vi "FTW-Container-Object-FromContainer.vi"(0 "FTW-Container In":variant, 11 "error in":errorcluster) -> (6 "?":T1, 15 "error out":errorcluster)   [LabVIEW 2015, in "FTW-Container.lvclass"]
uses:
  FTW-Container.lvclass
  FTW-Container-Object.ctl
  <vilib>/Utility/Data Type/NI_Data Type.lvlib
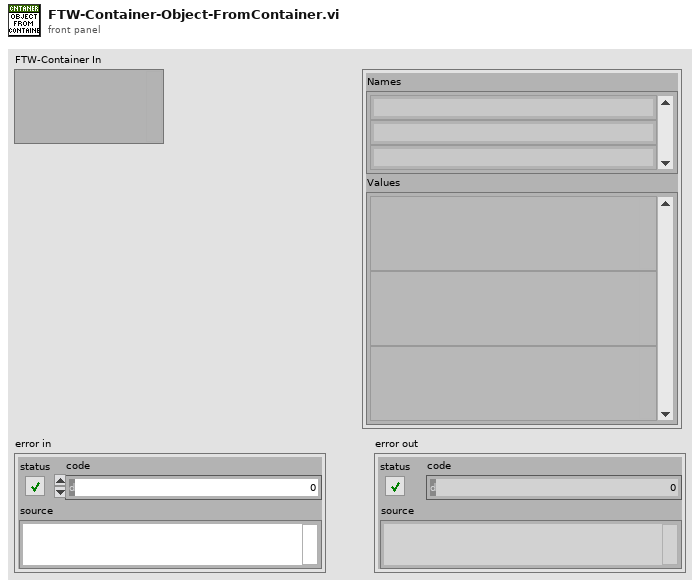
[diagram p1: front panel]
types:
  T1 = typedef "FTW-Container.lvclass/FTW-Container-Object.ctl" = cluster{"Names":string[], "Values":variant[]}
  T2 = typedef "NI_Data Type.lvlib/Data Type.ctl" = enum8{"Invalid Type", "Void", "I8", "I16", "I32", "I64", "U8", "U16", "U32", "U64", "Single Float", "Double Float", "Extended Float", "Single Complex", "Double Complex", "Extended Complex", "Enum U8", "Enum U16", "Enum U32", "Enum U64", "Single Float With Unit", "Double Float With Unit", "Extended Float With Unit", "Single Complex with Unit", "Double Complex with Unit", "Extended Complex with Unit", "Boolean", "String", "Path", "Picture", "Tag", "Array", "Cluster", "Variant", "LV Variant", "Waveform", "Timestamp", "Digital Waveform", "Digital Data", "ExpressData", "Refnum", "External Data", "VI", "Poly VI", "LabVIEW Class Instance", "Fixed Point"}
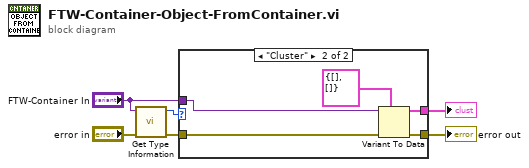
[diagram p0: block diagram]
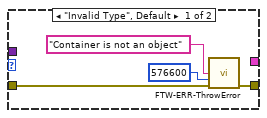
[diagram p2: hidden frame]
diagram:
  n1 = call <vilib>:"Get Type Information.vi"("error in (no error)"="error in", "Variant"="FTW-Container In") -> ("error out"=w4:errorcluster, "Type"=w2:T2)  [unwired: 5 in, 3 out]
  n2 = case shown="\"Cluster\"" w2 {
    tunnel: w4 -> [w10 w15]
    tunnel: [w9 w13] -> w3
    tunnel: "FTW-Container In" -> [_ w14]
    tunnel: [_ w11] -> w1
    frame "Invalid Type", Default {
      n3 = call "FTW-ERR-ThrowError.vi"("Error Message"="Container is not an object", "Error Code"=576600, "error in"=w10) -> ("error out"=w9:errorcluster)  [unwired: 12 in]
    }
    frame "Cluster" {
      n4 = Variant To Data(error in=w15, type=T1 {"Names"=[], "Values"=[]} ("Object"), Variant=w14) -> (data=w11:T1, error out=w13:errorcluster)
    }
  }
  "error out" <- w3
  "?" <- w1
